vi "lvHistoricalQuery.vi"(0 "Path to Python.exe":path=path "C:/ProgramData/Anaconda3/python.exe", 2 "startTime":string, 3 "endTime":string, 5 "error in (no error)":errorcluster, 7 "gaugeselection":bool[](array[boolean]), 8 "Path":path, 9 "SaveData":bool, 11 "tcselection":bool[](array[boolean])) -> (14 "Raw Python String Output":string, 19 "error out":errorcluster)   [LabVIEW 2017]
panel:
  out "Standard Error":string
  out "Return Code":i32
  # "1. Inputs - Set before running VI"
  # "2. Outputs"
  # "3. Errors - Both Standard and LabVIEW"
  # "A + B ="
  # "This VI sends inputs to a simple Python script, and returns its output.\n\nSee block diagram for code and comments"
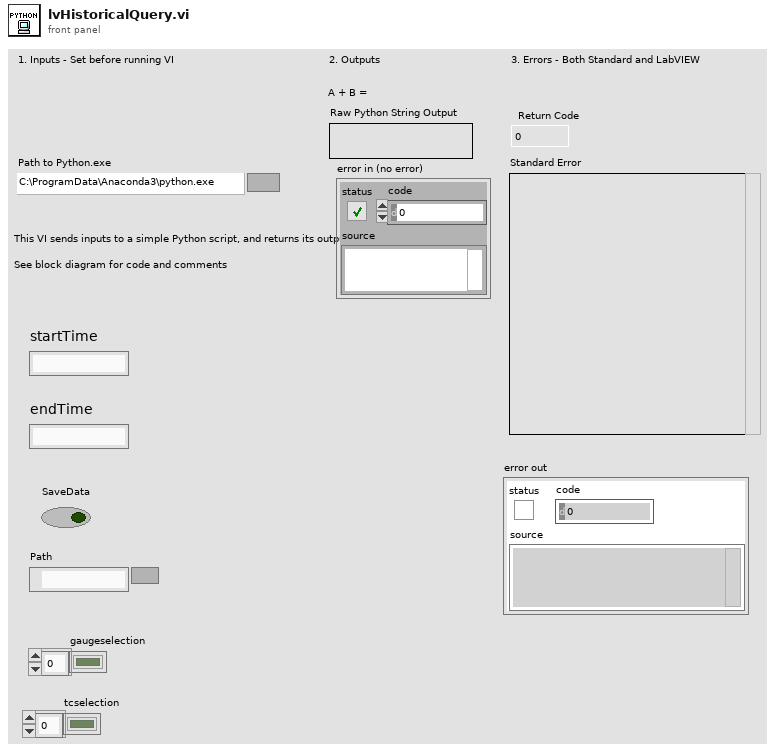
[diagram p1: front panel]
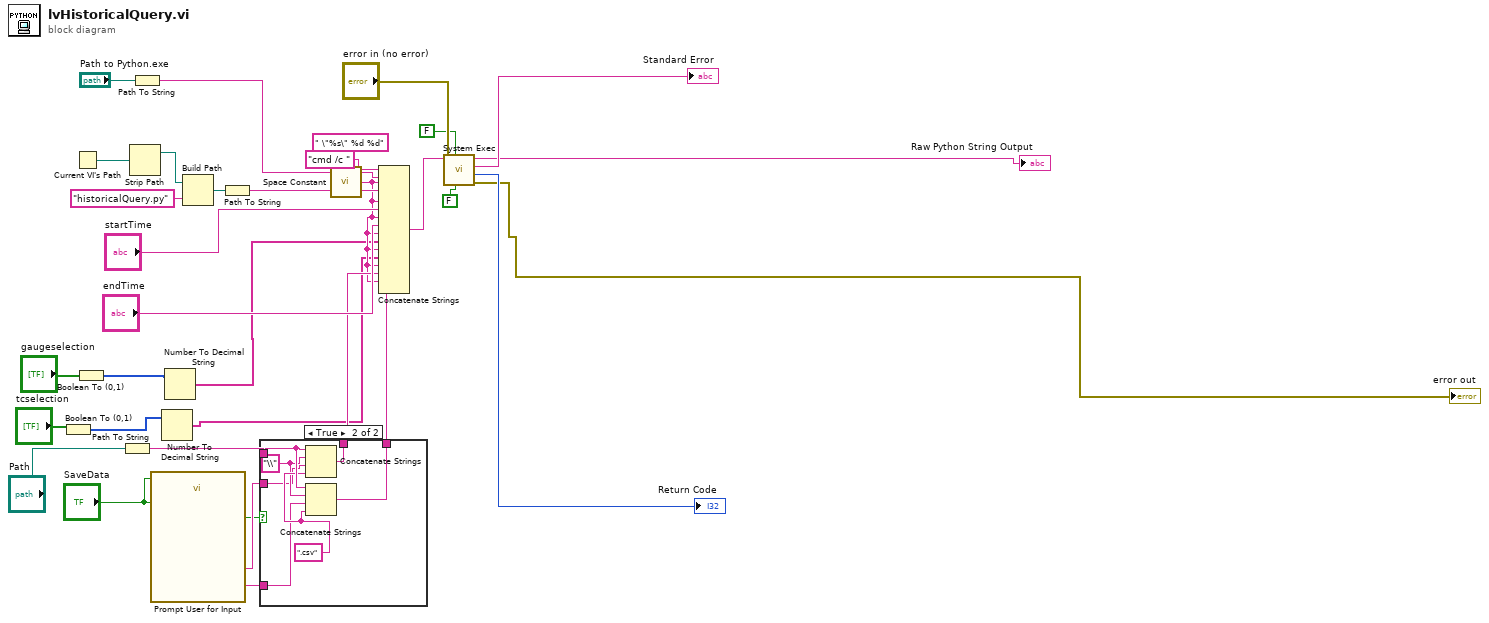
[diagram p0: block diagram]
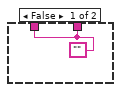
[diagram p2: hidden frame]
diagram:
  (unwired) " \"%s\" %d %d" ("format string")
  n1 = Boolean To (0,1)(Boolean="tcselection") -> (0, 1=w3:i16[])
  n2 = Current VI's Path() -> (path=w27:path)
  n3 = Boolean To (0,1)(Boolean="gaugeselection") -> (0, 1=w4:i16[])
  n4 = Path To String(path="Path") -> (string=w14:string)
  n5 = Strip Path(path=w27) -> (stripped path=w25:path)  [unwired: 1 out]
  n6 = Path To String(path="Path to Python.exe") -> (string=w22:string)
  n7 = call "Prompt User for Input"("Enable"="SaveData") -> ("Filename for Pressure"=w11:string, "Filename for Temperatures"=w12:string)  [unwired: 15 in, 2 out]
  n8 = Number To Decimal String(number=w3) -> (decimal integer string=w1:string[])  [unwired: 1 in]
  n9 = Number To Decimal String(number=w4) -> (decimal integer string=w2:string[])  [unwired: 1 in]
  n10 = Build Path(base path=w25, name or relative path="historicalQuery.py" ("Path to Function")) -> (appended path=w28:path)
  n11 = Path To String(path=w28) -> (string=w23:string)
  n12 = case shown="True" "SaveData" {
    tunnel: [w33 w40] -> w7
    tunnel: w14 -> [_ w39]
    tunnel: [w33 w38] -> w5
    tunnel: w12 -> [_ w35]
    tunnel: w11 -> [_ w34]
    frame False {
      w33 = ""
    }
    frame True {
      w37 = ".csv"
      w36 = "\\"
      n13 = Concatenate Strings(w39, w36, w35, w37) -> (w40:string)
      n14 = Concatenate Strings(w39, w36, w34, w37) -> (w38:string)
    }
  }
  n15 = call <vilib>:"Space Constant.vi"() -> ("String"=w6:string)
  n16 = Concatenate Strings("cmd /c " ("string"), w22, w6, w23, w6, "startTime", w6, "endTime", w6, w2, w6, w1, w6, w7, w6, w5) -> (w24:string)
  n17 = call <vilib>:"System Exec.vi"("run minimized? (F)"=FALSE, "wait until completion? (T)"=FALSE, "error in (no error)"="error in (no error)", "command line"=w24) -> ("error out"=→"error out":errorcluster, "return code"=→"Return Code":i32, "standard error"=→"Standard Error":string, "standard output"=→"Raw Python String Output":string)  [unwired: 4 in]
